vi "ErrorHandler.vi"(0 "Fehler (Eingang, kein Fehler)":errorcluster, 5 "instanceHandle":u32, 7 "DLL-Path":path, 9 "ERR_CODE":i32) -> (4 "Fehler (Ausgang)":errorcluster, 6 "instanceHandle":u32, 8 "DLL-Path":path, 10 "errText":string)   [LabVIEW 2015, in "MEDAQLib.lvlib"]
doc: "Sub-VI that returns an extended error message to the error code of a MedaQLib Sub-VI."
uses:
  MEDAQLib.lvlib
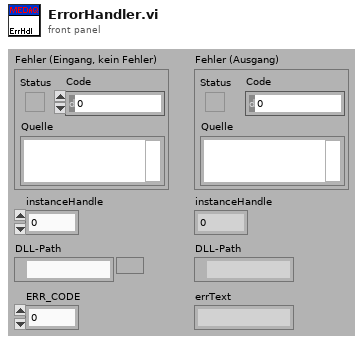
[diagram p1: front panel]
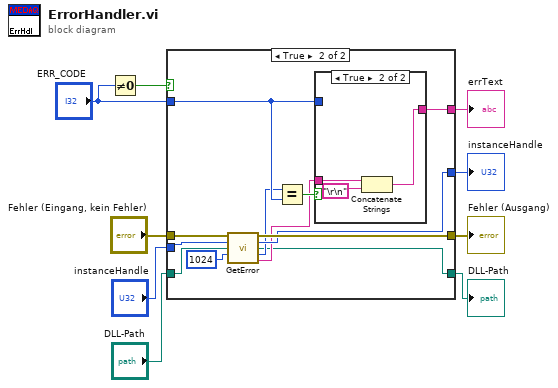
[diagram p0: block diagram]
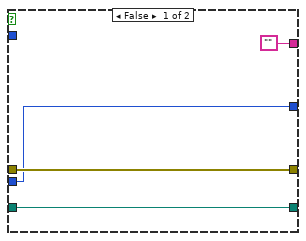
[diagram p2: hidden frame]
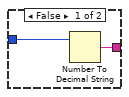
[diagram p3: hidden frame]
diagram:
  n1 = Not Equal To 0?(x="ERR_CODE") -> (x != 0?=w7:bool)
  n2 = case shown="True" w7 {
    tunnel: "Fehler (Eingang, kein Fehler)" -> [w13 w22]
    tunnel: "instanceHandle" -> [w11 w20]
    tunnel: [w13 w19] -> w9
    tunnel: ["" w24] -> w5
    tunnel: [w11 w18] -> w4
    tunnel: "ERR_CODE" -> [_ w23]
    tunnel: [w10 w15] -> w2
    tunnel: "DLL-Path" -> [w10 w14]
    frame False {
    }
    frame True {
      n3 = call "GetError.vi"("Fehler (Eingang, kein Fehler)"=w22, "instanceHandle"=w20, "DLL-Path"=w14, "maxLen"=u32 1024) -> ("Fehler (Ausgang)"=w19:errorcluster, "instanceHandle"=w18:u32, "DLL-Path"=w15:path, "ERR_CODE"=w17:i32, "errText"=w16:string)  [unwired: 7 out]
      n4 = Equal?(x=w17, y=w23) -> (x = y?=w25:bool)
      n5 = case shown="True" w25 {
        tunnel: w16 -> [_ w29]
        tunnel: [w27 w28] -> w24
        tunnel: w23 -> [w26 _]
        frame False {
          n6 = Number To Decimal String(number=w26) -> (decimal integer string=w27:string)  [unwired: 1 out]
        }
        frame True {
          n7 = Concatenate Strings(w29, "\r\n") -> (w28:string)
        }
      }
    }
  }
  "errText" <- w5
  "instanceHandle" <- w4
  "DLL-Path" <- w2
  "Fehler (Ausgang)" <- w9
